vi "sub_ReadPhotoR_Lin.vi"(7 "Paired R (10kO)":dbl=10000.0, 8 "error in":errorcluster, 9 "Analog Input Pin (0)":u8, 10 "vcc (5V)":dbl=5.0, 11 "Arduino Resource":T1={"VISA resource"="", "Board Type"=enum."Uno", "Connection Type"=enum."USB / Serial", "Bytes Per Packet (15)"=15}) -> (0 "error out":errorcluster, 2 "Intesity":dbl, 3 "Arduino Resource 2":T1={"VISA resource"="", "Board Type"=enum."Uno", "Connection Type"=enum."USB / Serial", "Bytes Per Packet (15)"=15})   [LabVIEW 2019]
uses:
  <vilib>/LabVIEW Interface for Arduino/Type Defs/Arduino Resource.ctl
  <vilib>/LabVIEW Interface for Arduino/Type Defs/Board Type.ctl
  <vilib>/LabVIEW Interface for Arduino/LabVIEW Interface for Arduino.lvlib
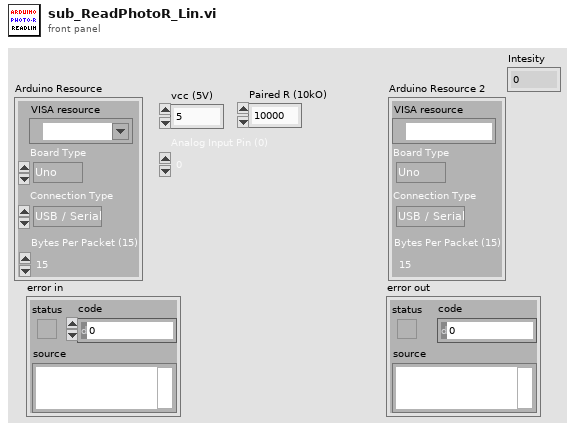
[diagram p1: front panel]
types:
  T1 = typedef "LabVIEW Interface for Arduino.lvlib/Arduino Resource.ctl" = cluster{"VISA resource":refnum<visa-resource-name>, "Board Type":T2, "Connection Type":enum8{"USB / Serial"}, "Bytes Per Packet (15)":u8}
  T2 = typedef "LabVIEW Interface for Arduino.lvlib/Board Type.ctl" = enum16{"Uno", "Dimuelanove w/Atmega 328", "Mega 2560"}
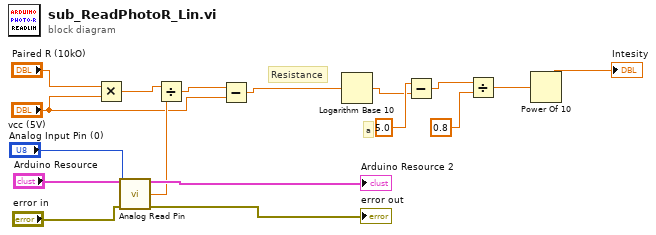
[diagram p0: block diagram]
diagram:
  # "a"
  # "Resistance"
  n1 = Multiply(x="Paired R (10kO)", y="vcc (5V)") -> (x*y=w11:dbl)
  n2 = call <vilib>:"Analog Read Pin.vi"("Arduino Resource"="Arduino Resource", "Analog Input Pin (0)"="Analog Input Pin (0)", "error in"="error in") -> ("Arduino Resource"=→"Arduino Resource 2":T1, "Voltage"=w10:dbl, "error out"=→"error out":errorcluster)  [unwired: 10 in]
  n3 = Divide(x=w11, y=w10) -> (x/y=w9:dbl)
  n4 = Subtract(x=w9, y="vcc (5V)") -> (x-y=w7:dbl)
  n5 = Logarithm Base 10(1:w7) -> (0:w1:dbl)
  n6 = Subtract(x=5.0 ("y"), y=w1) -> (x-y=w5:dbl)
  n7 = Divide(x=w5, y=0.8) -> (x/y=w4:dbl)
  n8 = Power Of 10(x=w4) -> (10^x=→"Intesity":dbl)
